vi "json_test_write.vi"(11 "Application Directory":path) -> ()   [LabVIEW 2020]
uses:
  Globals/FPGA Globals.vi
panel:
  out "JSON string":string
  in  "Adapter Module 2":enum16{"5772-DC", "5772-AC"}(ring)
  in  "Controls":T1={"Use FlexRIO Trigger"=TRUE, "RIO Resource Name"="", "Use detected RIO resource"=FALSE, "Ethernet Card WinPCap Port "=0, "FPGA Card"="", "Adapter Module"=""}
  out "Detected RIO Resource Name":string
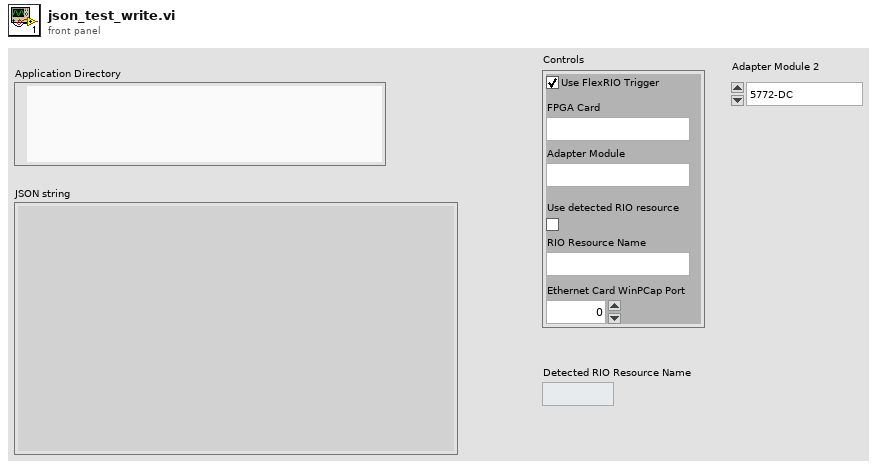
[diagram p1: front panel]
types:
  T1 = cluster{"Use FlexRIO Trigger":bool, "RIO Resource Name":string, "Use detected RIO resource":bool, "Ethernet Card WinPCap Port ":i16, "FPGA Card":string, "Adapter Module":string}
  T2 = enum16{"open", "replace", "create", "open or create", "replace or create", "replace or create with confirmation"}
  T3 = cluster{"Adapter Module":enum16{"5772-DC", "5772-AC"}, "FPGA Card":enum16{"7976R", "7975R"}, "Use FlexRIO Trigger":bool, "RIO Resource Name":string, "Use detected RIO resource":bool, "Ethernet Card WinPCap Port ":i16}
  T4 = typedef "FPGA_DAQ_settings.ctl" = cluster{"Use FlexRIO Trigger":bool, "RIO Resource Name":string, "Use detected RIO resource":bool, "Ethernet Card WinPCap Port ":i16, "Adapter Module":T5, "FPGA Card":T6}
  T5 = typedef "FPGA_adapter_type.ctl" = enum16{"5772-DC", "5772-AC"}
  T6 = typedef "FPGA_card_type.ctl" = enum16{"7976R", "7975R", "7966R"}
  T7 = enum32{"invalid app kind", "Development System", "Run Time System", "Student Edition", "Embedded LabVIEW", "Evaluation", "Custom"}
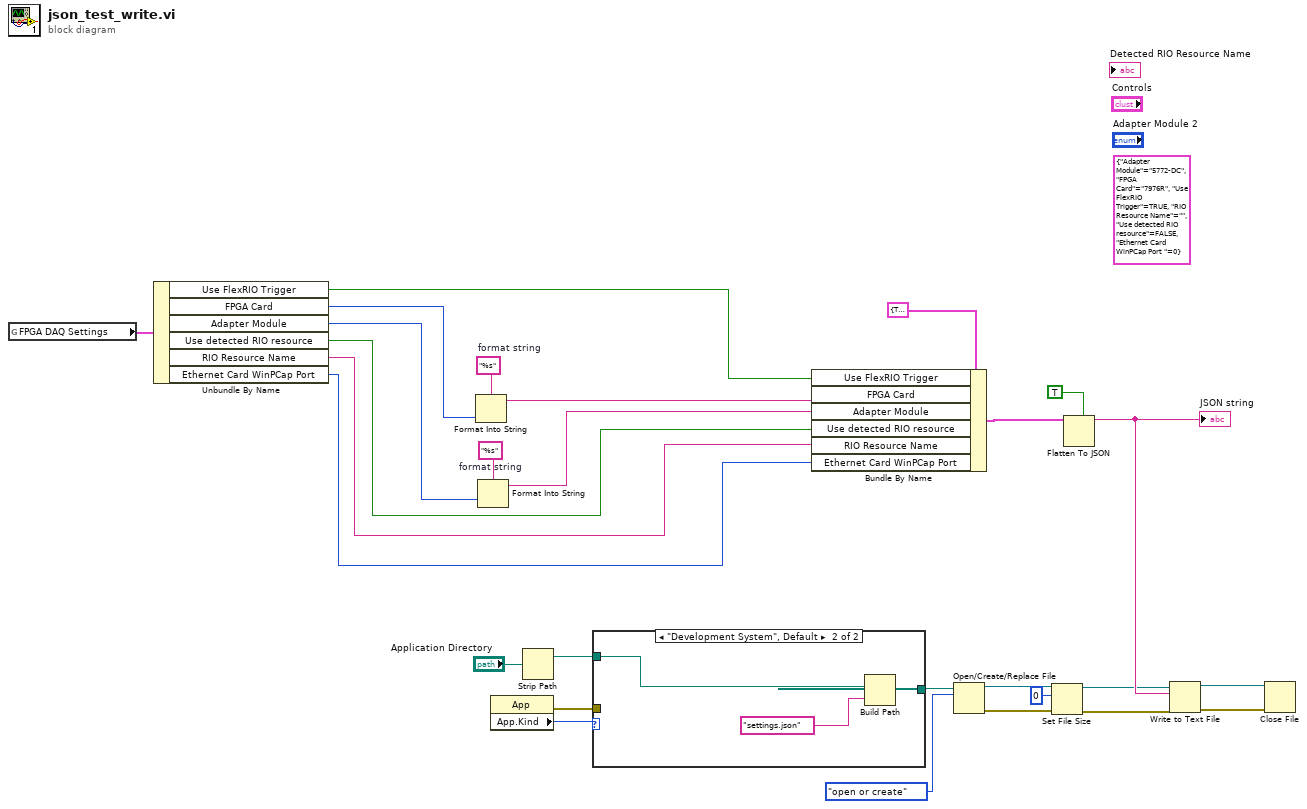
[diagram p0: block diagram]
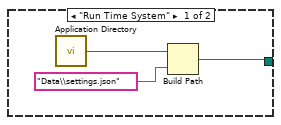
[diagram p2: hidden frame]
diagram:
  w24 = "%s"  # format string
  w26 = "%s"  # format string
  (unwired) T3 {"Adapter Module"=enum."5772-DC", "FPGA Card"=enum."7976R", "Use FlexRIO Trigger"=TRUE, "RIO Resource Name"="", "Use detected RIO resource"=FALSE, "Ethernet Card WinPCap Port "=0} ("Controls 2")
  n1 = global read "FPGA Globals.vi" "FPGA DAQ Settings"() -> (w9:T4)
  n2 = Unbundle By Name(w9) -> ("Use FlexRIO Trigger"=w8:bool, "FPGA Card"=w7:T6, "Adapter Module"=w6:T5, "Use detected RIO resource"=w5:bool, "RIO Resource Name"=w4:string, "Ethernet Card WinPCap Port"=w3:i16)
  n3 = Format Into String "Format Into String"(format string=w26, w7) -> (resulting string=w25:string)  [unwired: 2 in, 1 out]
  n4 = Format Into String "Format Into String"(format string=w24, w6) -> (resulting string=w23:string)  [unwired: 2 in, 1 out]
  n5 = property class="App"() -> (error out=w11:errorcluster, "App.Kind"=w12:T7)  [unwired: 2 in, 1 out]
  n6 = Strip Path(path="Application Directory") -> (stripped path=w1:path)  [unwired: 1 out]
  n7 = case shown="\"Development System\", Default" w12 {
    tunnel: [w29 w33] -> w10
    tunnel: w11 -> [_ _]
    tunnel: w1 -> [_ w32]
    frame "Run Time System" {
      n8 = call <vilib>:"Application Directory.vi"() -> ("Application Directory"=w31:path)
      n9 = Build Path(base path=w31, name or relative path="Data\\settings.json") -> (appended path=w29:path)
    }
    frame "Development System", Default {
      n10 = Build Path(base path=w32, name or relative path="settings.json") -> (appended path=w33:path)
    }
  }
  n11 = Bundle By Name(cluster=T1 {"Use FlexRIO Trigger"=TRUE, "RIO Resource Name"="", "Use detected RIO resource"=FALSE, "Ethernet Card WinPCap Port "=0, "FPGA Card"="", "Adapter Module"=""} ("Controls 2"), "Use FlexRIO Trigger"=w8, "FPGA Card"=w25, "Adapter Module"=w23, "Use detected RIO resource"=w5, "RIO Resource Name"=w4, "Ethernet Card WinPCap Port"=w3) -> (w28:T1)
  n12 = Open/Create/Replace File(file path (use dialog)=w10, operation (0:open)=T2."open or create") -> (refnum out=w15:refnum<file>, error out=w17:errorcluster)  [unwired: 4 in, 1 out]
  n13 = Set File Size(4:w17, 6:i64 0 ("size (in bytes)"), 7:w15) -> (0:w16:errorcluster, 3:w14:refnum<file>)
  n14 = Flatten To JSON(enable LabVIEW extensions? (T)=TRUE, anything=w28) -> (JSON string=w21:string)  [unwired: 1 in, 1 out]
  "JSON string" <- w21
  n15 = Write to Text File(file (use dialog)=w14, text=w21, error in=w16) -> (refnum out=w19:refnum<file>, error out=w20:errorcluster)  [unwired: 1 in, 1 out]
  n16 = Close File(refnum=w19, error in=w20) -> ()  [unwired: 2 out]
